vi "Pokayoke_no_List.vi"(8 "error in (no error)":errorcluster, 9 "Table Name":string, 10 "Part Number":string, 11 "Refnum in":T1) -> (0 "error out":errorcluster, 2 "Pokayoke List":string[](array[string]), 3 "Refnum out":T1)   [LabVIEW 2020]
uses:
  <vilib>/addons/database/Connection.llb/Conn ObjectReference.ctl
  <vilib>/addons/database/_DB Variant To Data/Database Variant To Data.xnode
  <vilib>/addons/database/NI_Database_API.lvlib
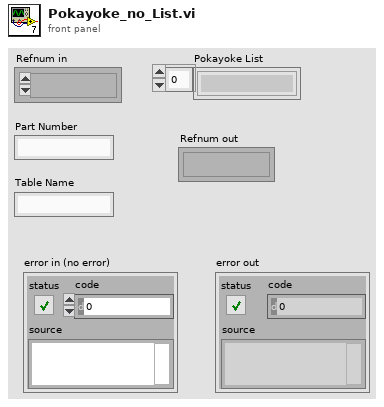
[diagram p1: front panel]
types:
  T1 = typedef "NI_Database_API.lvlib/Conn ObjectReference.ctl" = refnum<k1>
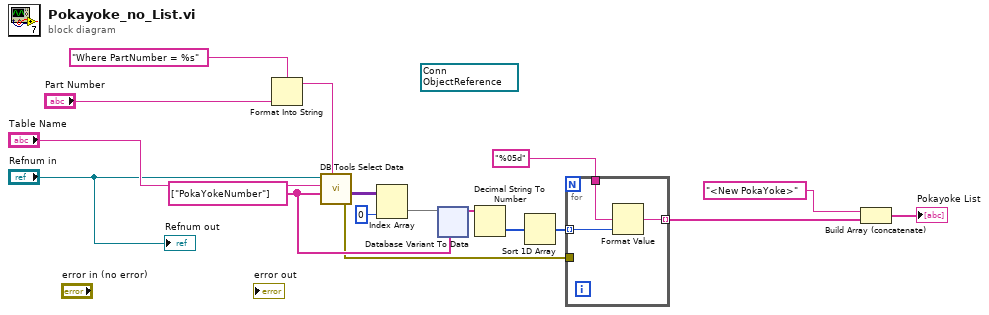
[diagram p0: block diagram]
diagram:
  (unwired) T1 refnum items=["Connection"] ("Refnum out")
  w12 = string[] ["PokaYokeNumber"] ("columns")
  n1 = Format Into String(format string="Where PartNumber = %s" ("String"), "Part Number") -> (resulting string=w6:string)  [unwired: 2 in, 1 out]
  n2 = call <vilib>:"DB Tools Select Data.vi"("condition"=w6, "columns"=w12, "table"="Table Name", "connection reference"="Refnum in") -> ("error out"=w2:errorcluster, "data"=w8:variant[][])  [unwired: 2 in, 1 out]
  n3 = Index Array(array=w8, index (col)=0 ("disabled index (col)")) -> (element=w11:variant[])  [unwired: 1 in]
  n4 = xnode "Database Variant To Data"("database variant"=w11, "type"=w12) -> ("data"=w14:string[])  [unwired: 1 in, 1 out]
  n5 = Decimal String To Number(string=w14) -> (number=w13:i32[])  [unwired: 2 in, 1 out]
  n6 = Sort 1D Array(array=w13) -> (sorted array=w15:i32[])
  n7 = for {
    tunnel: w15 -> [w20] mode=indexing
    tunnel: [w19] -> w16 mode=indexing
    tunnel: "%05d" ("format string") -> [w18]
    tunnel: w2 -> [_]
    n8 = Format Value(format string=w18, value (0)=w20) -> (output string=w19:string)  [unwired: 1 in]
  }
  n9 = Build Array (concatenate)("<New PokaYoke>" ("String"), w16) -> (→"Pokayoke List":string[])
  "Refnum out" <- "Refnum in"
